vi "SendMessageToAll.vi"(8 "error in (no error)":errorcluster, 9 "message value":variant, 10 "message name":string, 11 "Qbus in":refnum<class "Qbus.lvclass">) -> (0 "error in (no error)":errorcluster, 3 "Qbus out":refnum<class "Qbus.lvclass">)   [LabVIEW 2017, in "Qbus.lvclass"]
uses:
  <vilib>/addons/Qbus/Qbus.lvclass
  <vilib>/addons/Qbus/controls/message.ctl
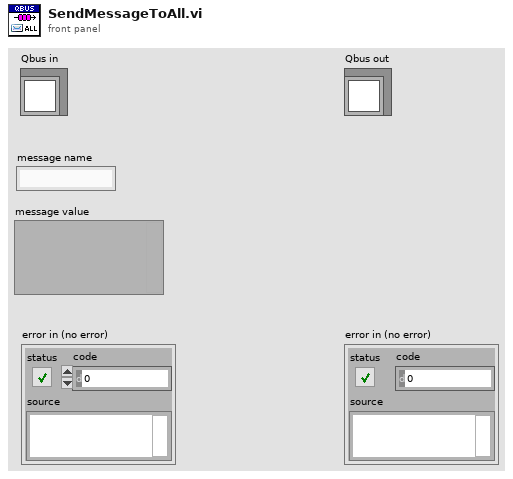
[diagram p1: front panel]
types:
  T1 = typedef "Qbus.lvclass/message.ctl" = cluster{"MsgName":string, "MsgValue":variant}
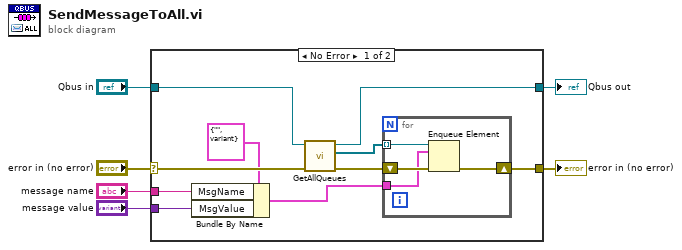
[diagram p0: block diagram]
diagram:
  n1 = case shown="No Error" "error in (no error)" {
    selector: "error in (no error)" -> [w16 w22]
    tunnel: [w11 w22] -> w5
    tunnel: [w14 w21] -> w3
    tunnel: "Qbus in" -> [w15 w21]
    tunnel: "message name" -> [w8 _]
    tunnel: "message value" -> [w7 _]
    frame No Error {
      n2 = Bundle By Name(cluster=T1 {"MsgName"="", "MsgValue"=variant} ("Message"), "MsgName"=w8, "MsgValue"=w7) -> (w10:T1)
      n3 = call <vilib>:"GetAllQueues.vi"("error in (no error)"=w16, "Qbus in"=w15) -> ("error in (no error)"=w13:errorcluster, "queues"=w12:refnum<queue>[], "Qbus out"=w14:refnum<class "Qbus.lvclass">)  [unwired: 7 in]
      n4 = for {
        shift-right: [w18] -> w11
        shift-left: w13 -> [w20]
        tunnel: w12 -> [w19] mode=indexing
        tunnel: w10 -> [w17]
        n5 = Enqueue Element(queue=w19, element=w17, error in (no error)=w20) -> (error out=w18:errorcluster)  [unwired: 1 in, 2 out]
      }
    }
    frame Error {
    }
  }
  "error in (no error)" <- w5
  "Qbus out" <- w3
